vi "Dequeue Trace (Testing Only).vi"(8 "error in (no error)":errorcluster, 9 "timeout in ms (-1)":i32, 11 "AF Trace Queue in":refnum<class "AF Trace Queue.lvclass">) -> (0 "error out":errorcluster, 1 "timed out?":bool, 2 "Trace String":string, 3 "AF Trace Queue out":refnum<class "AF Trace Queue.lvclass">)   [LabVIEW 2020, in "AF Trace Queue.lvclass"]
uses:
  AF Trace Queue.lvclass
  AF Trace Queue.lvclass/AF Trace Queue.ctl
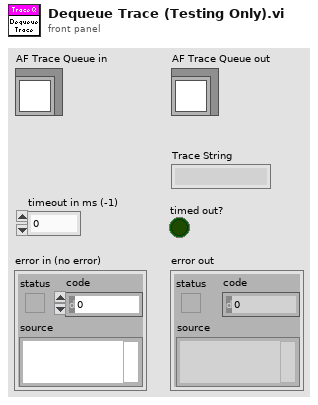
[diagram p1: front panel]
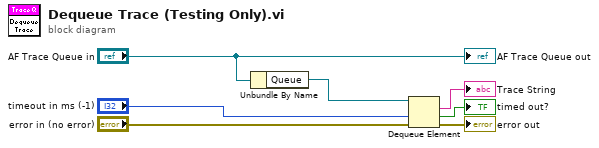
[diagram p0: block diagram]
diagram:
  n1 = Unbundle By Name("AF Trace Queue in") -> ("Queue"=w6:refnum<queue>)
  n2 = Dequeue Element(queue=w6, timeout in ms (-1)="timeout in ms (-1)", error in (no error)="error in (no error)") -> (element=→"Trace String":string, timed out?=→"timed out?":bool, error out=→"error out":errorcluster)  [unwired: 1 out]
  "AF Trace Queue out" <- "AF Trace Queue in"
